vi "Filtering_2011.vi"(4 "Filters":cluster{"Name":string, "#Filters":dbl}[](array[cluster])) -> (1 "Filter factor":dbl)   [LabVIEW 2020]
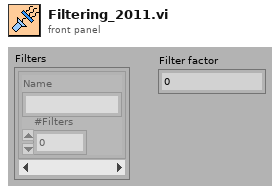
[diagram p1: front panel]
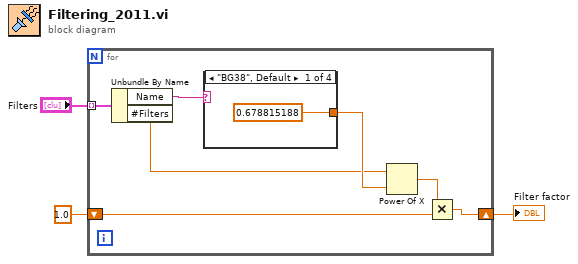
[diagram p0: block diagram]
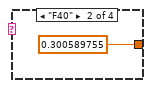
[diagram p2: hidden frame]
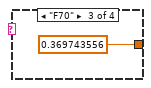
[diagram p3: hidden frame]
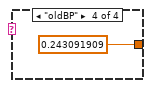
[diagram p4: hidden frame]
diagram:
  n1 = for {
    tunnel: "Filters" -> [w10] mode=indexing
    shift-right: [w4] -> w3
    shift-left: 1.0 -> [w5]
    n2 = Unbundle By Name(w10) -> ("Name"=w9:string, "#Filters"=w7:dbl)
    n3 = case shown="\"BG38\", Default" w9 {
      tunnel: [0.678815188 0.300589755 0.369743556 0.243091909] -> w8
      frame "BG38", Default {
      }
      frame "F40" {
      }
      frame "F70" {
      }
      frame "oldBP" {
      }
    }
    n4 = Power Of X(1:w8, 2:w7) -> (0:w6:dbl)
    n5 = Multiply(x=w6, y=w5) -> (x*y=w4:dbl)
  }
  "Filter factor" <- w3
